vi "PCO_GetCameraRamSize.vi"(8 "error in (no error)":errorcluster {"code" format="%x"}, 11 "ph":u64) -> (0 "error out":errorcluster {"code" format="%x"}, 1 "dwRamSize":u32, 2 "ErrorMessage":i32 format="%x", 3 "ph out":u64, 5 "wPageSize":u16)   [LabVIEW 2019, in "SDK.lvlib" / "StorageControl.lvlib"]
doc: "<b>Description:</b>\nThis function returns the size of the camera internal memory in CamRAM pages and the CamRAM page size in pixels.\n\n<b>Supported camera type:</b>\npco.dimax, pco.1200, pco.1600, pco.2000, pco.4000\n\n<b>Descriptor dependency:</b>\ndwGeneralCapsDESC1: NO_RECORDER"
uses:
  StorageControl.lvlib
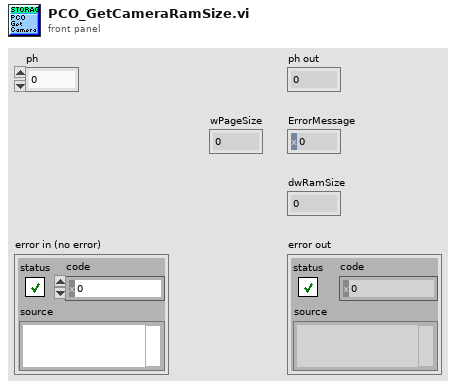
[diagram p1: front panel]
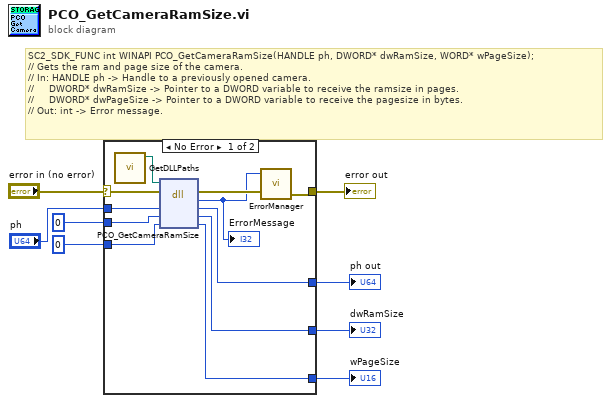
[diagram p0: block diagram]
diagram:
  # "SC2_SDK_FUNC int WINAPI PCO_GetCameraRamSize(HANDLE ph, DWORD* dwRamSize, WORD* wPageSize);\n// Gets the ram and page size of the camera.\n// In: HANDLE ph -> Handle to a previously opened camera.\n//     DWORD* dwRamSize -> Pointer to a DWORD variable to receive the ramsize in pages.\n//     DWORD* dwPageSize -> Pointer to a DWORD variable to receive the pagesize in bytes.\n// Out: int -> Error message."
  n1 = case shown="No Error" "error in (no error)" {
    selector: "error in (no error)" -> [w13 w23]
    tunnel: "ph" -> [w19 w22]
    tunnel: [w18 w22] -> w7
    tunnel: u32 0 ("dwRamSize") -> [w17 w21]
    tunnel: [w16 w21] -> w5
    tunnel: u16 0 ("wPageSize") -> [w15 w20]
    tunnel: [w14 w20] -> w3
    tunnel: [w11 w23] -> w2
    frame No Error {
      n2 = call "GetDLLPaths.vi"() -> ("SC2_Cam_Path"=w9:path)  [unwired: 8 in, 3 out]
      n3 = dll-call lib="?" fn="PCO_GetCameraRamSize"(path in=w9, error in=w13, "ph"=w19, "dwRamSize"=w17, "wPageSize"=w15) -> (error out=w12:errorcluster, "return type"=w10:i32, "ph"=w18:u64, "dwRamSize"=w16:u32, "wPageSize"=w14:u16)  [unwired: 1 in, 1 out]
      "ErrorMessage" <- w10
      n4 = call "ErrorManager.vi"("error in (no error)"=w12, "error code"=w10) -> ("error out"=w11:errorcluster)  [unwired: 2 in, 1 out]
    }
    frame Error {
    }
  }
  "ph out" <- w7
  "dwRamSize" <- w5
  "wPageSize" <- w3
  "error out" <- w2
